vi "AIT 429 Initialization VI.vi"(8 "error in (no error)":errorcluster, 10 "Custom XML":string, 11 "Device Item Ref in":T1 format="%.0x") -> (0 "error out":errorcluster, 3 "Device Item Ref out":T1 format="%.0x")   [LabVIEW 2015, in "AIT 429 System Explorer.lvlib"]
uses:
  <vilib>/NI Veristand/Custom Device API/Custom Device Item Ref.ctl
  <vilib>/NI Veristand/Custom Device API/Custom Device Channel.ctl
  <vilib>/NI Veristand/Custom Device API/Custom Device Channel Type.ctl
  Shared/Controls and Global/Global.vi
  AIT 429 System Explorer.lvlib
  <vilib>/NI Veristand/Custom Device API/Custom Device API.lvlib
  Shared/AIT 429 Shared.lvlib
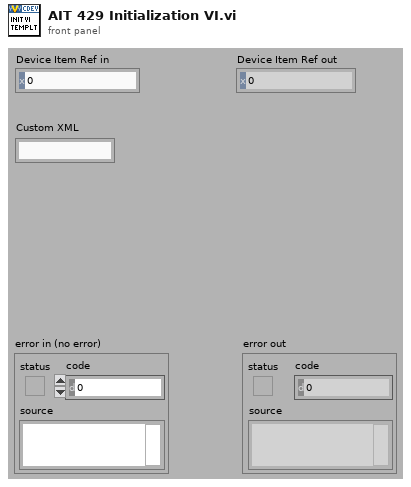
[diagram p1: front panel]
types:
  T1 = typedef "Custom Device API.lvlib/Custom Device Item Ref.ctl" = u64
  T2 = typedef "Custom Device API.lvlib/Custom Device Channel.ctl" = cluster{"Type":T3, "Units":string, "Default Value":dbl, "Faultable":bool, "Scalable":bool}
  T3 = typedef "Custom Device API.lvlib/Custom Device Channel Type.ctl" = enum16{"Input", "Output"}
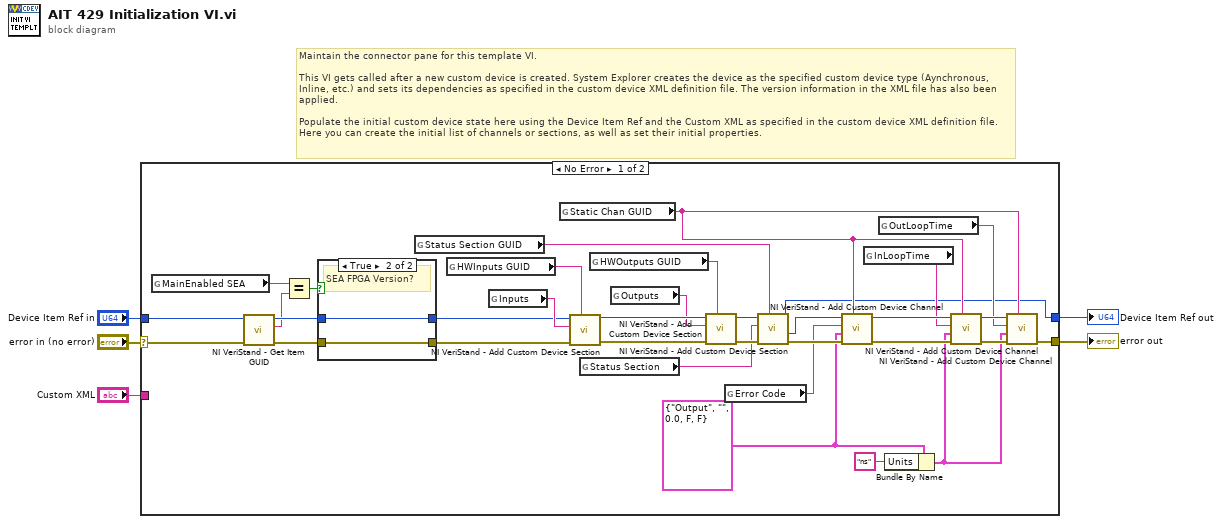
[diagram p0: block diagram]
diagram:
  # "Maintain the connector pane for this template VI.\n\nThis VI gets called after a new custom device is created. System Explorer creates the device as the specified custom device type (Aynchronous, Inline, etc.) and sets its dependencies as specified in the custom device XML definition file. The version information in the XML file has also been applied.\n\nPopulate the initial custom device state here using the Device Item Ref and the Custom XML as specified in the custom device XML definition file. Here you can create the initial list of channels or sections, as well as set their initial properties."
  n1 = case shown="No Error" "error in (no error)" {
    selector: "error in (no error)" -> [w13 w45]
    tunnel: [w17 w44] -> w4
    tunnel: "Device Item Ref in" -> [w14 w44]
    tunnel: "Custom XML" -> [_ _]
    tunnel: [w18 w45] -> w1
    frame No Error {
      w19 = T2 {"Type"=enum."Output", "Units"="", "Default Value"=0.0, "Faultable"=FALSE, "Scalable"=FALSE} ("Channel")
      n2 = global read "Global.vi" "MainEnabled SEA"() -> (w12:string)
      n3 = call <vilib>:"NI VeriStand - Get Item GUID.vi"("error in (no error)"=w13, "Item Ref in"=w14) -> ("error out"=w9:errorcluster, "GUID"=w6:string, "Item Ref out"=w10:T1)  [unwired: 7 in]
      n4 = Equal?(x=w12, y=w6) -> (x = y?=w11:bool)
      n5 = case shown="True" w11 {
        tunnel: w10 -> [w41 w43]
        tunnel: w9 -> [w40 w42]
        tunnel: [w41 w43] -> w8
        tunnel: [w40 w42] -> w7
        frame False {
        }
        frame True {
          # "SEA FPGA Version?"
        }
      }
      n6 = global read "Global.vi" "Status Section GUID"() -> (w29:string)
      n7 = global read "Global.vi" "HWInputs GUID"() -> (w35:string)
      n8 = global read "Global.vi" "Inputs"() -> (w37:string)
      n9 = global read "Global.vi" "Static Chan GUID"() -> (w20:string)
      n10 = call <vilib>:"NI VeriStand - Add Custom Device Section.vi"("GUID (Default Section)"=w35, "error in (no error)"=w7, "Section Name"=w37, "Parent Ref in"=w8) -> ("error out"=w39:errorcluster, "Parent Ref out"=w38:T1)  [unwired: 4 in, 2 out]
      n11 = global read "Global.vi" "Status Section"() -> (w27:string)
      n12 = global read "Global.vi" "HWOutputs GUID"() -> (w34:string)
      n13 = global read "Global.vi" "Outputs"() -> (w36:string)
      n14 = call <vilib>:"NI VeriStand - Add Custom Device Section.vi"("GUID (Default Section)"=w34, "error in (no error)"=w39, "Section Name"=w36, "Parent Ref in"=w38) -> ("error out"=w33:errorcluster, "Parent Ref out"=w32:T1)  [unwired: 4 in, 2 out]
      n15 = global read "Global.vi" "Error Code"() -> (w28:string)
      n16 = call <vilib>:"NI VeriStand - Add Custom Device Section.vi"("GUID (Default Section)"=w29, "error in (no error)"=w33, "Section Name"=w27, "Parent Ref in"=w32) -> ("error out"=w31:errorcluster, "Section Ptr"=w30:T1, "Parent Ref out"=w17:T1)  [unwired: 4 in, 1 out]
      n17 = call <vilib>:"NI VeriStand - Add Custom Device Channel.vi"("GUID (Default Channel)"=w20, "error in (no error)"=w31, "Channel"=w19, "Channel Name"=w28, "Parent Ref in"=w30) -> ("error out"=w26:errorcluster, "Parent Ref out"=w24:T1)  [unwired: 3 in, 2 out]
      n18 = global read "Global.vi" "InLoopTime"() -> (w22:string)
      n19 = global read "Global.vi" "OutLoopTime"() -> (w21:string)
      n20 = Bundle By Name(cluster=w19, "Units"="ns") -> (w16:T2)
      n21 = call <vilib>:"NI VeriStand - Add Custom Device Channel.vi"("GUID (Default Channel)"=w20, "error in (no error)"=w26, "Channel"=w16, "Channel Name"=w22, "Parent Ref in"=w24) -> ("error out"=w25:errorcluster, "Parent Ref out"=w23:T1)  [unwired: 3 in, 2 out]
      n22 = call <vilib>:"NI VeriStand - Add Custom Device Channel.vi"("GUID (Default Channel)"=w20, "error in (no error)"=w25, "Channel"=w16, "Channel Name"=w21, "Parent Ref in"=w23) -> ("error out"=w18:errorcluster)  [unwired: 3 in, 3 out]
    }
    frame Error {
    }
  }
  "error out" <- w1
  "Device Item Ref out" <- w4
